vi "MachineStates.vi"() -> ()   [LabVIEW 2019]
panel:
  out "NextState":T1(ring)
  in  "MachineStates":T1(ring)
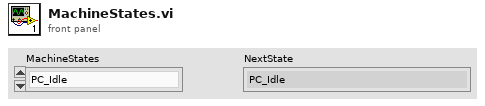
[diagram p1: front panel]
types:
  T1 = enum16{"PC_Idle", "Part_Load", "Part_Presence_Check", "Door_Closed", "LoadCellCalibration", "ServoMoveToApproachPosition", "ServoMoveToTargetPosition", "ServoMoveToHomePosition", "Doors_Open"}
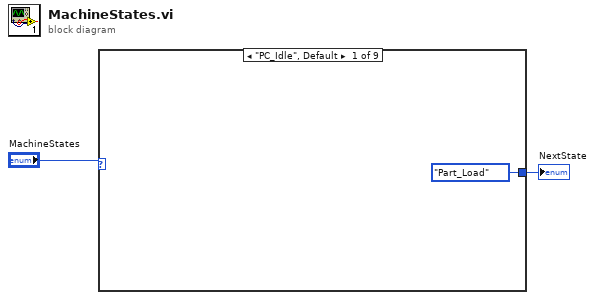
[diagram p0: block diagram]
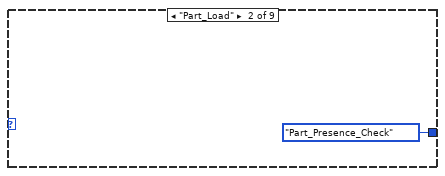
[diagram p2: hidden frame]
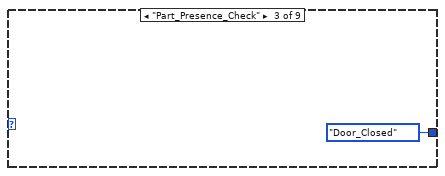
[diagram p3: hidden frame]
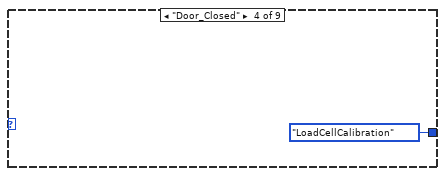
[diagram p4: hidden frame]
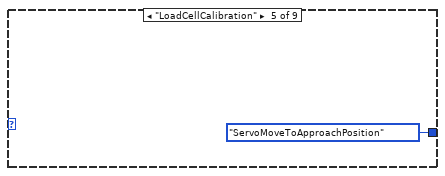
[diagram p5: hidden frame]
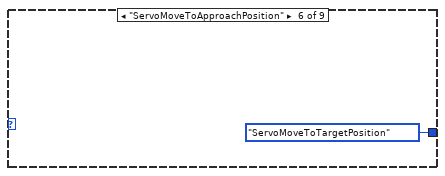
[diagram p6: hidden frame]
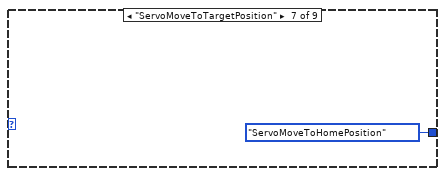
[diagram p7: hidden frame]
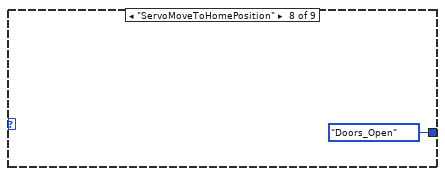
[diagram p8: hidden frame]
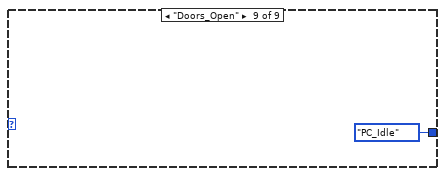
[diagram p9: hidden frame]
diagram:
  n1 = case shown="\"PC_Idle\", Default" "MachineStates" {
    tunnel: [T1."Part_Load" ("Enum") T1."Part_Presence_Check" ("Enum") T1."Door_Closed" ("Enum") T1."LoadCellCalibration" ("Enum") T1."ServoMoveToApproachPosition" ("Enum") T1."ServoMoveToTargetPosition" ("Enum") T1."ServoMoveToHomePosition" ("Enum") T1."Doors_Open" ("Enum") T1."PC_Idle" ("Enum")] -> w1
    frame "PC_Idle", Default {
    }
    frame "Part_Load" {
    }
    frame "Part_Presence_Check" {
    }
    frame "Door_Closed" {
    }
    frame "LoadCellCalibration" {
    }
    frame "ServoMoveToApproachPosition" {
    }
    frame "ServoMoveToTargetPosition" {
    }
    frame "ServoMoveToHomePosition" {
    }
    frame "Doors_Open" {
    }
  }
  "NextState" <- w1
